vi "plot_data_update_matrixUpdate.vi"(0 "XY plot":i32[][](array[numeric]), 3 "idx Y":i32, 5 "idx X":i32, 8 "Y size":i32) -> (11 "In Range?":bool, 14 "XY plot out":i32[][](array[numeric]), 17 "idx Y out":i32)   [LabVIEW 2010, in "OSA.lvclass"]
doc: "SubVI to a <B>Thorlabs_OSA_32</B> object.\n\n[GOOP 1.0]"
uses:
  OSA.lvclass
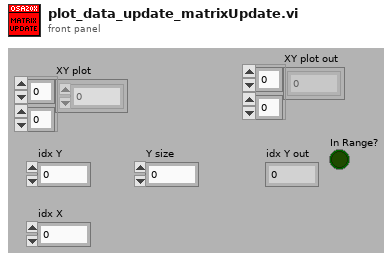
[diagram p1: front panel]
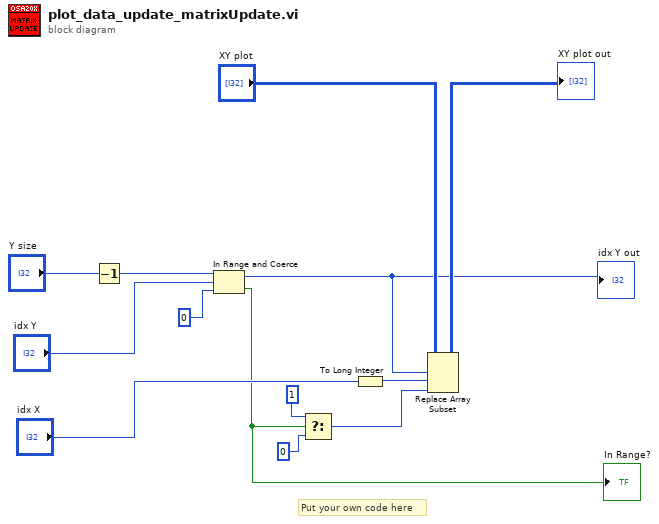
[diagram p0: block diagram]
diagram:
  # "Put your own code here"
  n1 = Decrement(x="Y size") -> (x-1=w7:i32)
  n2 = In Range and Coerce(upper limit=w7, x="idx Y", lower limit=0) -> (coerced(x)=w5:i32, In Range?=w4:bool)
  "idx Y out" <- w5
  "In Range?" <- w4
  n3 = Select(t=1 ("new element/subarray"), s=w4, f=0) -> (s? t:f=w1:i32)
  n4 = To Long Integer(number="idx X") -> (32bit integer=w13:i32)
  n5 = Replace Array Subset(array="XY plot", new element=w1, index (row)=w5, index (col)=w13) -> (→"XY plot out":i32[][])
